vi "AAA Charger_Catalog.vi"   [LabVIEW 2020]
uses:
  Charger_Next_Action.ctl
  Charger_States_Control.ctl
  Charger_Status Refnum.ctl
panel:
  # "Charger Catalog"
types:
  T1 = typedef "Charger_Status Refnum.ctl" = refnum<vi>
  T2 = typedef "Semaphore RefNum" = refnum<k1>
  T3 = typedef "Charger_Next_Action.ctl" = cluster{"ChargingState":string, "Temp":enum16{"Any", "GT 3", "LE 3", "GT 2", "LE 2"}, "Low Limit":dbl, "High Limit":dbl, "Charger":T4, "Adjustment":dbl}
  T4 = typedef "Charger_States_Control.ctl" = enum16{"Enable", "Disable", "Adjust", "Pause", "na"}
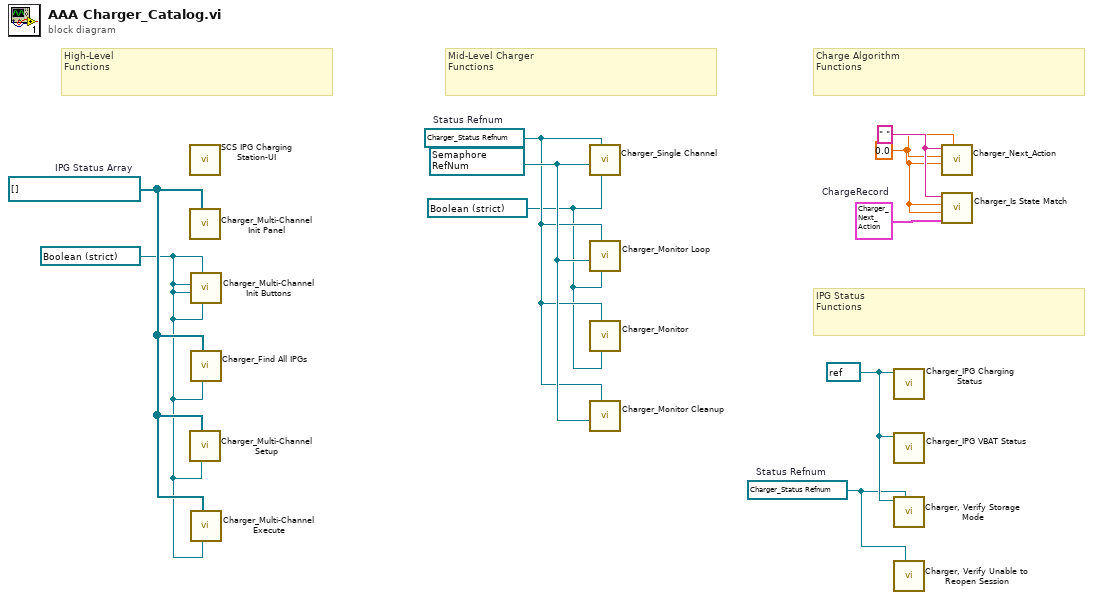
[diagram p0: block diagram]
diagram:
  w1 = T1 refnum  # Status Refnum
  w2 = refnum<visa-resource-name> refnum ("MICS Dongle Address")
  w7 = T2 refnum items=["semaphore"] ("semaphore")
  w4 = refnum<vi> refnum ("button refnum")
  w5 = T1 refnum  # Status Refnum
  w6 = T1[] []  # IPG Status Array
  w3 = refnum<vi> refnum ("button refnum")
  w9 = T3 {"ChargingState"="CHARGE_PRE_CONDITION-1", "Temp"=enum."LE 3", "Low Limit"=-inf, "High Limit"=225.0, "Charger"=enum."Adjust", "Adjustment"=-100.0}  # ChargeRecord
  w8 = 0.0 ("Temperature")
  w10 = " " ("ChargingState")
  # "IPG Status\nFunctions"
  # "Charge Algorithm\nFunctions"
  # "Mid-Level Charger\nFunctions"
  # "High-Level\nFunctions"
  n1 = call "SCS IPG Charging Station-UI.vi"() -> ()  [unwired: 12 in]
  n2 = call "Charger_Multi-Channel Init Panel.vi"("Status Refnum  Array"=w6) -> ()  [unwired: 8 in, 1 out]
  n3 = call "Charger_Multi-Channel Setup.vi"("STOP Refnum"=w3, "Status Refnum  Array"=w6) -> ()  [unwired: 9 in, 1 out]
  n4 = call "Charger_Multi-Channel Init Buttons.vi"("STOP refnum"=w3, "RUN refnum"=w3, "PRINT refnum"=w3, "VBAT refnum"=w3) -> ()  [unwired: 7 in, 1 out]
  n5 = call "Charger_Find All IPGs.vi"("Stop Refnum"=w3, "IPG Status Array"=w6) -> ()  [unwired: 9 in, 1 out]
  n6 = call "Charger_Multi-Channel Execute.vi"("STOP Refnum"=w3, "Status Refnum  Array"=w6) -> ()  [unwired: 9 in, 1 out]
  n7 = call "Charger_Single Channel.vi"("Stop Refnum"=w4, "Status Refnum"=w5, "semaphore"=w7) -> ()  [unwired: 8 in, 1 out]
  n8 = call "Charger_Monitor Loop.vi"("Stop Refnum"=w4, "Status Refnum"=w5, "semaphore"=w7) -> ()  [unwired: 7 in, 2 out]
  n9 = call "Charger_Monitor.vi"("Stop Refnum"=w4, "Status Refnum"=w5) -> ()  [unwired: 8 in, 2 out]
  n10 = call "Charger_Monitor Cleanup.vi"("Status Refnum"=w5, "semaphore"=w7) -> ()  [unwired: 6 in, 2 out]
  n11 = call "Charger_IPG Charging Status.vi"("MICS Dongle Address"=w2) -> ()  [unwired: 7 in, 4 out]
  n12 = call "Charger_IPG VBAT Status.vi"("MICS Dongle Address"=w2) -> ()  [unwired: 8 in, 3 out]
  n13 = call "Charger, Verify Storage Mode.vi"("VISA resource"=w2, "Status Refnum"=w1) -> ()  [unwired: 7 in, 2 out]
  n14 = call "Charger, Verify Unable to Reopen Session.vi"("Status Refnum"=w1) -> ()  [unwired: 9 in, 1 out]
  n15 = call "Charger_Next_Action.vi"("Setpoint"=w8, "ReceivedLevel"=w8, "Temperature"=w8, "ChargingState"=w10) -> ()  [unwired: 2 in, 4 out]
  n16 = call "Charger_Is State Match.vi"("ChargeRecord"=w9, "ReceivedLevel"=w8, "TemperatureLevel"=w8, "ChargingState"=w10) -> ()  [unwired: 1 out]
